vi "perform fault handling.vi"(0 "module in":refnum<class "TBM module execution interface.lvclass">, 1 "module ref in":refnum<data-value>, 3 "error in":errorcluster, 4 "fault handling in":T4, 5 "run flags in":u8, 6 "fault fifo":refnum<k33>, 7 "engine error in":errorcluster, 8 "worker pool in":T1, 9 "cfg ref":refnum<data-value>, 11 "engine reference":i32, 12 "iteration":u64) -> (13 "engine error out":errorcluster, 14 "module out":refnum<class "TBM module execution interface.lvclass">, 15 "go to safe state":bool, 17 "error out":errorcluster, 19 "run flags out":u8)   [LabVIEW 2013, in "main engine.lvlib"]
uses:
  main engine/main engine.lvlib
  fault handling spec.ctl
  Configuration/Error Actions.ctl
  rt fault.ctl
  <vilib>/NI/Tag Bus Module Framework/runtime/error classification.ctl
  <vilib>/NI/Tag Bus Module Framework/module configuration/TBM module configuration.lvclass
  <vilib>/NI/Tag Bus Module Framework/runtime/TBM module execution interface.lvclass
  worker library/worker comms.ctl
  worker library/worker commands.ctl
  worker library/request fifos.ctl
  worker library/recovery request.ctl
  worker library/response fifos.ctl
  worker library/recovery response.ctl
  worker library/worker pool.lvlib
  Configuration/Standard Engine Configuration.lvclass
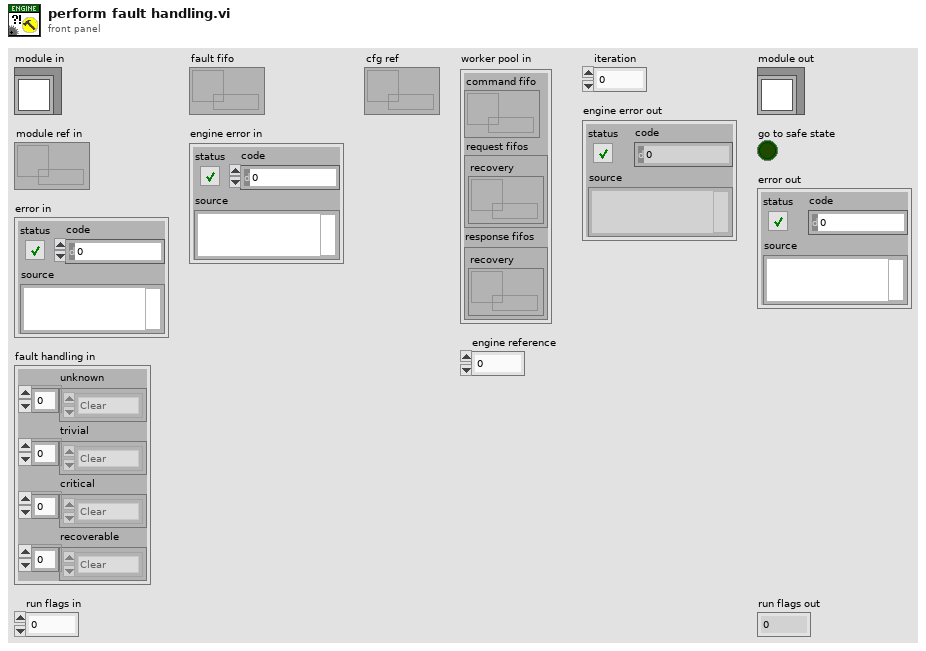
[diagram p1: front panel]
types:
  T1 = typedef "worker pool.lvlib/worker comms.ctl" = cluster{"command fifo":refnum<k33>, "request fifos":T2, "response fifos":T3}
  T2 = typedef "worker pool.lvlib/request fifos.ctl" = cluster{"recovery":refnum<k33>}
  T3 = typedef "worker pool.lvlib/response fifos.ctl" = cluster{"recovery":refnum<k33>}
  T4 = typedef "main engine.lvlib/fault handling spec.ctl" = cluster{"unknown":T5[], "trivial":T5[], "critical":T5[], "recoverable":T5[]}
  T5 = typedef "Standard Engine Configuration.lvclass/Error Actions.ctl" = enum16{"Clear", "Notify", "Stop Component", "Stop Engine", "Safe State", "Attempt Recovery"}
  T6 = typedef "TBM module execution interface.lvclass/error classification.ctl" = enum16{"unknown", "none", "trivial", "recoverable", "critical"}
  T7 = typedef "main engine.lvlib/rt fault.ctl" = cluster{"code":i32, "classification":T6, "iteration":u64, "cfg ref":refnum<data-value>}
  T8 = typedef "worker pool.lvlib/recovery request.ctl" = cluster{"module ref":refnum<data-value>, "engine reference":i32, "original run flags":u8, "attempts allowed":u16, "cfg ref":refnum<data-value>}
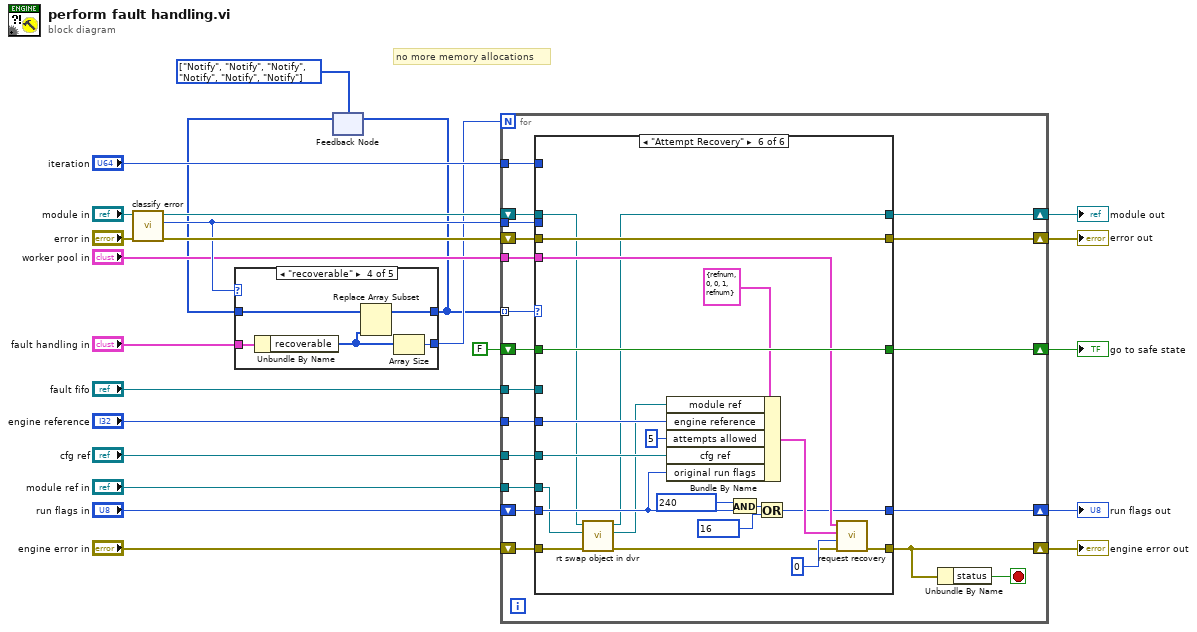
[diagram p0: block diagram]
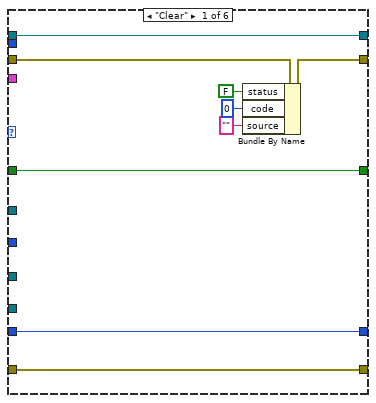
[diagram p2: hidden frame]
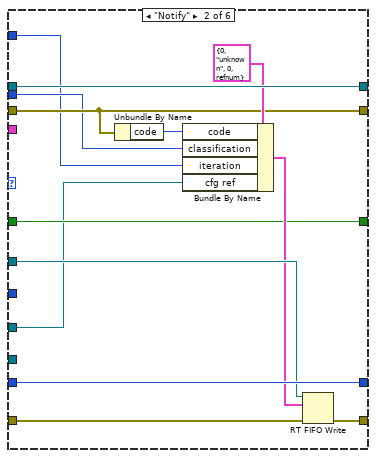
[diagram p3: hidden frame]
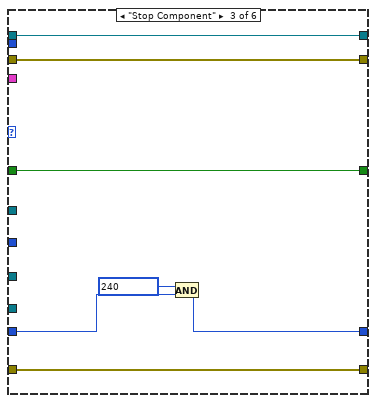
[diagram p4: hidden frame]
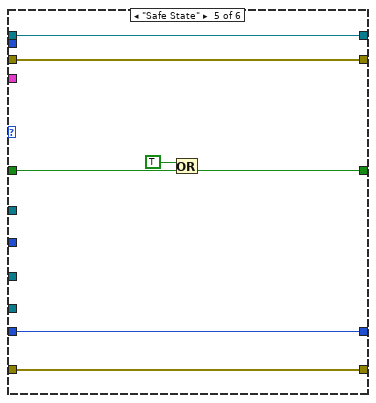
[diagram p6: hidden frame]
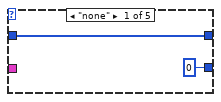
[diagram p7: hidden frame]
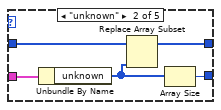
[diagram p8: hidden frame]
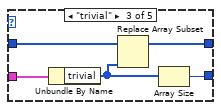
[diagram p9: hidden frame]
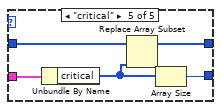
[diagram p10: hidden frame]
diagram:
  w1 = T5[] [enum."Notify", enum."Notify", enum."Notify", enum."Notify", enum."Notify", enum."Notify"] items=["Clear", "Notify", "Stop Component", "Stop Engine", "Safe State", "Attempt Recovery"] ("critical")
  # "no more memory allocations"
  n1 = call-dynamic "classify error.vi"("error to classify"="error in", "module in"="module in") -> ("classified error"=w19:errorcluster, "error classification"=w11:T6, "module out"=w18:refnum<class "TBM module execution interface.lvclass">)  [unwired: 7 in]
  n2 = feedback #1(w1) -> (w2:T5[])
  n3 = case shown="\"recoverable\"" w11 {
    tunnel: "fault handling in" -> [_ w31 w36 w41 w46]
    tunnel: [w25 w28 w33 w38 w43] -> w3
    tunnel: [0 w30 w35 w40 w45] -> w4
    tunnel: w2 -> [w25 w29 w34 w39 w44]
    frame "none" {
    }
    frame "unknown" {
      n4 = Unbundle By Name(w31) -> ("unknown"=w27:T5[])
      n5 = Replace Array Subset(array=w29, new element=w27) -> (w28:T5[])  [unwired: 1 in]
      n6 = Array Size(array=w27) -> (size(s)=w30:i32)
    }
    frame "trivial" {
      n7 = Unbundle By Name(w36) -> ("trivial"=w32:T5[])
      n8 = Replace Array Subset(array=w34, new element=w32) -> (w33:T5[])  [unwired: 1 in]
      n9 = Array Size(array=w32) -> (size(s)=w35:i32)
    }
    frame "recoverable" {
      n10 = Unbundle By Name(w41) -> ("recoverable"=w37:T5[])
      n11 = Replace Array Subset(array=w39, new element=w37) -> (w38:T5[])  [unwired: 1 in]
      n12 = Array Size(array=w37) -> (size(s)=w40:i32)
    }
    frame "critical" {
      n13 = Unbundle By Name(w46) -> ("critical"=w42:T5[])
      n14 = Replace Array Subset(array=w44, new element=w42) -> (w43:T5[])  [unwired: 1 in]
      n15 = Array Size(array=w42) -> (size(s)=w45:i32)
    }
  }
  n16 = feedback-in #1(w3) -> ()
  n17 = for {
    N: w4 -> [_]
    shift-right: [w58] -> w15
    shift-left: "run flags in" -> [w59]
    shift-right: [w61] -> w17
    shift-left: w19 -> [w62]
    shift-right: [w64] -> w16
    shift-left: w18 -> [w63]
    tunnel: "fault fifo" -> [w55]
    tunnel: w3 -> [w65] mode=indexing
    shift-right: [w56] -> w12
    shift-left: "engine error in" -> [w57]
    tunnel: w11 -> [w54]
    tunnel: "iteration" -> [w53]
    shift-right: [w52] -> w8
    shift-left: FALSE -> [w51]
    tunnel: "worker pool in" -> [w50]
    tunnel: "cfg ref" -> [w49]
    tunnel: "module ref in" -> [w60]
    tunnel: "engine reference" -> [w48]
    stop <- w47 stop-if-true
    n18 = case shown="\"Attempt Recovery\"" w65 {
      tunnel: [w74 w87 w94 w98 w105 w108] -> w64
      tunnel: w63 -> [w74 w87 w94 w98 w105 w109]
      tunnel: w62 -> [w73 w80 w93 w96 w104 w126]
      tunnel: [w70 w80 w93 w96 w104 w126] -> w61
      tunnel: w60 -> [_ _ _ _ _ w111]
      tunnel: w59 -> [w72 w86 w92 w97 w103 w114]
      tunnel: [w72 w86 w89 w97 w103 w117] -> w58
      tunnel: w57 -> [w71 w85 w91 _ w102 w107]
      tunnel: [w71 w84 w91 w96 w102 w123] -> w56
      tunnel: w55 -> [_ w83 _ _ _ _]
      tunnel: w54 -> [_ w78 _ _ _ _]
      tunnel: w53 -> [_ w77 _ _ _ _]
      tunnel: [w66 w76 w90 w95 w100 w125] -> w52
      tunnel: w51 -> [w66 w76 w90 w95 w101 w125]
      tunnel: w50 -> [_ _ _ _ _ w124]
      tunnel: w49 -> [_ w75 _ _ _ w113]
      tunnel: w48 -> [_ _ _ _ _ w115]
      frame "Clear" {
        n19 = Bundle By Name(cluster=w73, "status"=FALSE, "code"=0, "source"="") -> (w70:errorcluster)
      }
      frame "Notify" {
        n20 = Unbundle By Name(w80) -> ("code"=w79:i32)
        n21 = Bundle By Name(cluster=T7 {"code"=0, "classification"=enum."unknown", "iteration"=0, "cfg ref"=refnum} ("element"), "code"=w79, "classification"=w78, "iteration"=w77, "cfg ref"=w75) -> (w81:T7)
        n22 = RT FIFO Write(0:w83, 1:w81, 3:w85) -> (11:w84:errorcluster)  [unwired: 2 in, 3 out]
      }
      frame "Stop Component" {
        n23 = And(x=u8 240, y=w92) -> (x .and. y?=w89:u8)
      }
      frame "Stop Engine" {
        # "Passing an engine error out stops the engine."
      }
      frame "Safe State" {
        n24 = Or(x=TRUE, y=w101) -> (x .or. y?=w100:bool)
      }
      frame "Attempt Recovery" {
        n25 = call "rt swap object in dvr.vi"("error in"=w107, "module ref in in"=w111, "module in"=w109) -> ("error out"=w106:errorcluster, "module ref out"=w110:refnum<data-value>, "module out"=w108:refnum<class "TBM module execution interface.lvclass">)  [unwired: 6 in]
        n26 = Bundle By Name(cluster=T8 {"module ref"=refnum, "engine reference"=0, "original run flags"=0, "attempts allowed"=1, "cfg ref"=refnum} ("recovery request"), "module ref"=w110, "engine reference"=w115, "attempts allowed"=u16 5, "cfg ref"=w113, "original run flags"=w114) -> (w120:T8)
        n27 = And(x=u8 240, y=w114) -> (x .and. y?=w119:u8)
        n28 = Or(x=w119, y=u8 16 ("x")) -> (x .or. y?=w117:u8)
        n29 = call "request recovery.vi"("error in"=w106, "timeout in ms (0)"=0, "recovery request"=w120, "worker comms in"=w124) -> ("error out"=w123:errorcluster)  [unwired: 7 in]
      }
    }
    n30 = Unbundle By Name(w56) -> ("status"=w47:bool)
  }
  "error out" <- w17
  "module out" <- w16
  "run flags out" <- w15
  "engine error out" <- w12
  "go to safe state" <- w8
